vi "XIPIN_3GPP_Searcher_1_0.vi"   [LabVIEW 2017]
doc: "The 3GPP Searcher core is a highly integrated solution for identifying the multiple transmission paths of users in a 3GPP uplink. The core includes all the logic required for scramble code generation, correlation, accumulation and filtering in a single co-processor, easily integrated with a DSP or microprocessor.\n------------------------------------\n<b>Need License</b> : Yes"
uses:
  <vilib>/rvi/XilinxIP/XIPIN_XNode/niFpgaXIPIN.xnode
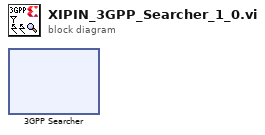
[diagram p0: block diagram]
diagram:
  n1 = xnode ("3GPP Searcher")() -> ()
